vi "Index.vi"(8 "error in (no error)":errorcluster, 10 "Index":i32, 11 "Time Stamp Array in":refnum<class "Time Stamp Array.lvclass">) -> (0 "error out":errorcluster, 3 "Indexed element":refnum<class "Generic Data.lvclass">)   [LabVIEW 2020, in "Data.lvlib" / "Time Stamp Array.lvclass"]
doc: "Index an element from 'Generic Data in'.\nThis implementation returns a generic Time Stamp class with the indexed Time Stamp."
uses:
  Time Stamp Array.lvclass
  Generic Data.lvclass
  Time Stamp Array.lvclass/Time Stamp Array.ctl
  Time Stamp/Time Stamp.lvclass/Time Stamp.ctl
  Time Stamp/Time Stamp.lvclass
  C:/Users/Henri/OneDrive/LabVIEW/Framework/Data/Generic Data/Generic Data.lvclass
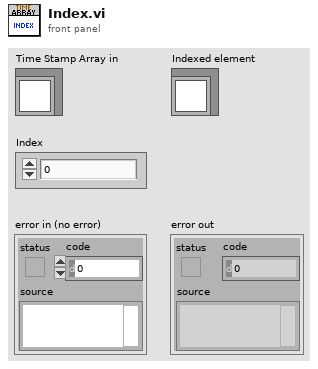
[diagram p1: front panel]
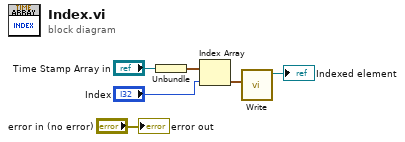
[diagram p0: block diagram]
diagram:
  n1 = Unbundle("Time Stamp Array in") -> (w5:timestamp[])
  n2 = Index Array(array=w5, index="Index") -> (element=w2:timestamp)
  n3 = call "Write.vi"("Time Stamp"=w2) -> ("Time Stamp out"=→"Indexed element":refnum<class "Time Stamp.lvclass">)  [unwired: 10 in]
  "error out" <- "error in (no error)"
